vi "PH_ForceSensor.set i Attr.vi"(0 "VI in":refnum<vi>, 5 "error in (no error)":errorcluster) -> (14 "VI out":refnum<vi>, 16 "i Attribute":T1, 19 "error out":errorcluster)   [LabVIEW 2014, in "PH_ForceSensor.lvlib"]
uses:
  PH_ForceSensor.lvlib
  PH_ForceSensor.i attribute.ctl
  PH_ForceSensor.GUI Refs.ctl
  PH_ForceSensor.Dataset.ctl
  PH_ForceSensor.Ranges.ctl
  CSCore/CSSystem/CSSystemLib/CSSystemLib.lvlib
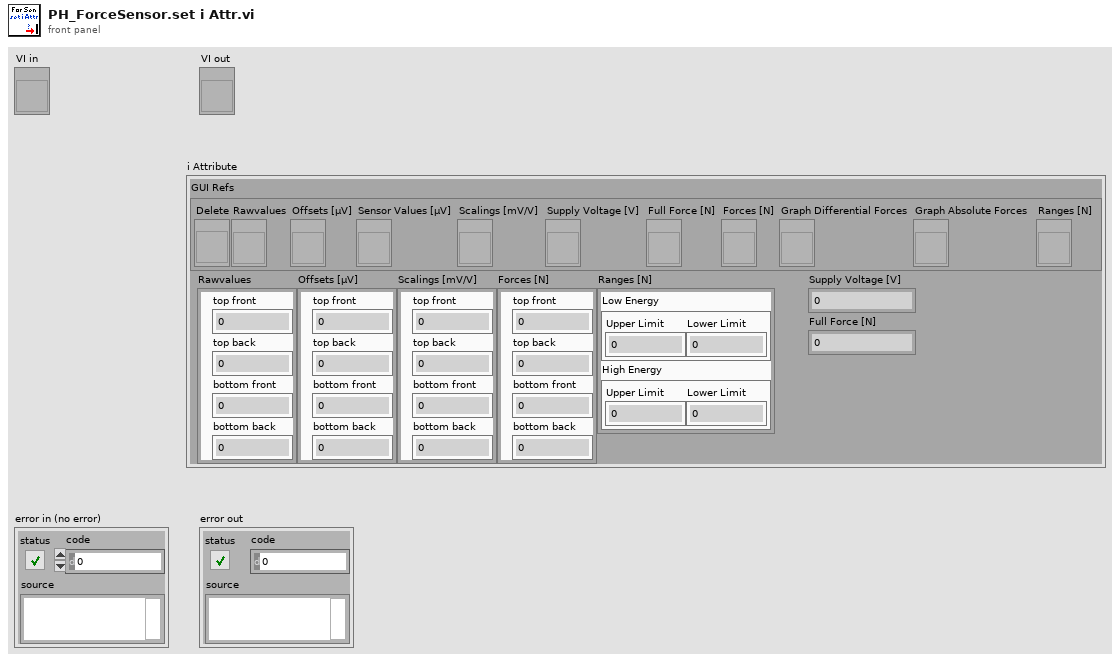
[diagram p1: front panel]
types:
  T1 = typedef "PH_ForceSensor.lvlib/PH_ForceSensor.i attribute.ctl" = cluster{"GUI Refs":T2, "Rawvalues":T3, "Offsets [µV]":T3, "Scalings [mV/V]":T3, "Forces [N]":T3, "Supply Voltage [V]":dbl, "Full Force [N]":dbl, "Ranges [N]":cluster{"Low Energy":cluster{"Upper Limit":dbl, "Lower Limit":dbl}, "High Energy":cluster{"Upper Limit":dbl, "Lower Limit":dbl}}}
  T2 = typedef "PH_ForceSensor.lvlib/PH_ForceSensor.GUI Refs.ctl" = cluster{"Delete":refnum<vi>, "Rawvalues":refnum<vi>, "Offsets [µV]":refnum<vi>, "Sensor Values [µV]":refnum<vi>, "Scalings [mV/V]":refnum<vi>, "Supply Voltage [V]":refnum<vi>, "Full Force [N]":refnum<vi>, "Forces [N]":refnum<vi>, "Graph Differential Forces":refnum<vi>, "Graph Absolute Forces":refnum<vi>, "Ranges [N]":refnum<vi>}
  T3 = typedef "PH_ForceSensor.lvlib/PH_ForceSensor.Dataset.ctl" = cluster{"top front":dbl, "top back":dbl, "bottom front":dbl, "bottom back":dbl}
  T4 = typedef "PH_ForceSensor.lvlib/PH_ForceSensor.Ranges.ctl" = cluster{"Low Energy":cluster{"Upper Limit":dbl, "Lower Limit":dbl}, "High Energy":cluster{"Upper Limit":dbl, "Lower Limit":dbl}}
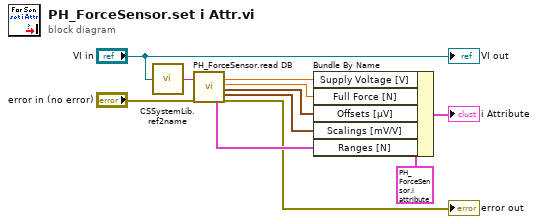
[diagram p0: block diagram]
diagram:
  n1 = call "CSSystemLib.ref2name.vi"("obj refnum"="VI in") -> ("name"=w8:string)
  n2 = call "PH_ForceSensor.read DB.vi"("Force Sensor Instance"=w8, "error in (no error)"="error in (no error)") -> ("Ranges [N]"=w3:T4, "Supply Voltage [V]"=w7:dbl, "Full Force [N]"=w6:dbl, "Offsets [µV]"=w5:T3, "Scalings [mV/V]"=w4:T3, "error out"=→"error out":errorcluster)  [unwired: 12 in]
  n3 = Bundle By Name(cluster=T1 {"GUI Refs"={"Delete"=refnum, "Rawvalues"=refnum, "Offsets [µV]"=refnum, "Sensor Values [µV]"=refnum, "Scalings [mV/V]"=refnum, "Supply Voltage [V]"=refnum, "Full Force [N]"=refnum, "Forces [N]"=refnum, "Graph Differential Forces"=refnum, "Graph Absolute Forces"=refnum, "Ranges [N]"=refnum}, "Rawvalues"={"top front"=0.0, "top back"=0.0, "bottom front"=0.0, "bottom back"=0.0}, "Offsets [µV]"={"top front"=0.0, "top back"=0.0, "bottom front"=0.0, "bottom back"=0.0}, "Scalings [mV/V]"={"top front"=0.0, "top back"=0.0, "bottom front"=0.0, "bottom back"=0.0}, "Forces [N]"={"top front"=0.0, "top back"=0.0, "bottom front"=0.0, "bottom back"=0.0}, "Supply Voltage [V]"=0.0, "Full Force [N]"=0.0, "Ranges [N]"={"Low Energy"={"Upper Limit"=0.0, "Lower Limit"=0.0}, "High Energy"={"Upper Limit"=0.0, "Lower Limit"=0.0}}} ("CLASS.i attribute"), "Supply Voltage [V]"=w7, "Full Force [N]"=w6, "Offsets [µV]"=w5, "Scalings [mV/V]"=w4, "Ranges [N]"=w3) -> (→"i Attribute":T1)
  "VI out" <- "VI in"
